vi "Capture and Playback Audio.vi"(10 "Feedback Event":refnum<user-event>, 11 "Command Queue":refnum<queue>) -> ()   [LabVIEW 2020]
uses:
  Controls/Latency Test Message.ctl
  Controls/Audio Device Refnum.ctl
  Controls/Latency Test Config.ctl
  Controls/Backends.ctl
  Controls/Latency Test Device Config.ctl
  Controls/Audio Device Config.ctl
  Controls/Audio Device Format.ctl
  Controls/Audio Device Advanced Config.ctl
  Controls/Latency Test Loopback State.ctl
  Controls/Audio Device Type.ctl
  Controls/Audio Device Info.ctl
  Controls/Audio Device Native Data Format.ctl
  888dee6f-a1d8-44b9-8463-aaa634a31580.vi
  afe3ba56-811c-4ec0-8caf-7165a7675817.vi
  Private/Result To Error.vi
  888dee6f-a1d8-44b9-8463-aaa634a31580.vi/6b901882-6109-4f44-aca5-48e1525e5248.vi
  888dee6f-a1d8-44b9-8463-aaa634a31580.vi/06c0137a-63d3-4e30-982f-115d83a1188c.vi
  Audio Devices/Get Audio Device Configuration.vi
  Private/Audio Device Refnum To Value.vi
  afe3ba56-811c-4ec0-8caf-7165a7675817.vi/4dfb5711-8d81-45a3-b3db-a84d40650863.vi
  afe3ba56-811c-4ec0-8caf-7165a7675817.vi/c8869513-30c6-44f2-a2d3-73232fe63870.vi
  888dee6f-a1d8-44b9-8463-aaa634a31580.vi/06c0137a-63d3-4e30-982f-115d83a1188c.vi/4b7b629c-2e91-4160-9820-a26af8f6e677.vi
  Private/ma_format To Audio Data Format.vi
  afe3ba56-811c-4ec0-8caf-7165a7675817.vi/4dfb5711-8d81-45a3-b3db-a84d40650863.vi/4b7b629c-2e91-4160-9820-a26af8f6e677.vi
  afe3ba56-811c-4ec0-8caf-7165a7675817.vi/c8869513-30c6-44f2-a2d3-73232fe63870.vi/4b7b629c-2e91-4160-9820-a26af8f6e677.vi
  <vilib>/Utility/Data Type/Get Numeric Information.vi
  <vilib>/Utility/error.llb/Error Cluster From Error Code.vi
  G-Audio.lvlib
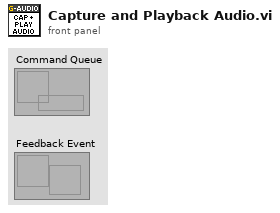
[diagram p1: front panel]
types:
  T1 = typedef "G-Audio.lvlib/Audio Device Refnum.ctl" = refnum<file>
  T2 = typedef "Latency Test Config.ctl" = cluster{"Backend":T3, "Read / Write Buffer":i32, "Capture Device":T4, "Playback Device":T4}
  T3 = typedef "G-Audio.lvlib/Backends.ctl" = enum16{"WASAPI", "DirectSound", "WinMM", "Core Audio", "sndio", "audio(4)", "OSS", "PulseAudio", "ALSA", "JACK", "AAudio", "OpenSL|ES", "Web Audio", "Custom", "Null", "Default"}
  T4 = typedef "Latency Test Device Config.ctl" = cluster{"Name":u16, "ID":u8[], "Buffer Size":u32, "Config":T5, "Advanced Config":T7}
  T5 = typedef "G-Audio.lvlib/Audio Device Config.ctl" = cluster{"Sample Rate (Hz)":u32, "Channels":u32, "Format":T6}
  T6 = typedef "G-Audio.lvlib/Audio Device Format.ctl" = enum16{"Native", "U8", "I16", "I32", "SGL"}
  T7 = typedef "G-Audio.lvlib/Audio Device Advanced Config.ctl" = cluster{"Exclusive Mode":bool, "Period Size":u32, "Num Periods":u32, "Optimize Latency":bool}
  T8 = typedef "Latency Test Loopback State.ctl" = enum16{"Idle", "Init", "Loopback", "Stop", "Shutdown", "Error"}
  T9 = typedef "Latency Test Message.ctl" = cluster{"Info":string, "Data":variant}
  T10 = typedef "G-Audio.lvlib/Audio Device Type.ctl" = enum16{"(None)", "Playback", "Capture", "Duplex", "Loopback"}
  T11 = typedef "G-Audio.lvlib/Audio Device Info.ctl" = cluster{"Name":string, "ID":u8[], "Device Type":T10, "Default":bool, "Native Data Formats":T12[]}
  T12 = typedef "G-Audio.lvlib/Audio Device Native Data Format.ctl" = cluster{"Format":T6, "Channels":u32, "Sample Rate (Hz)":u32, "Exclusive Mode":bool}
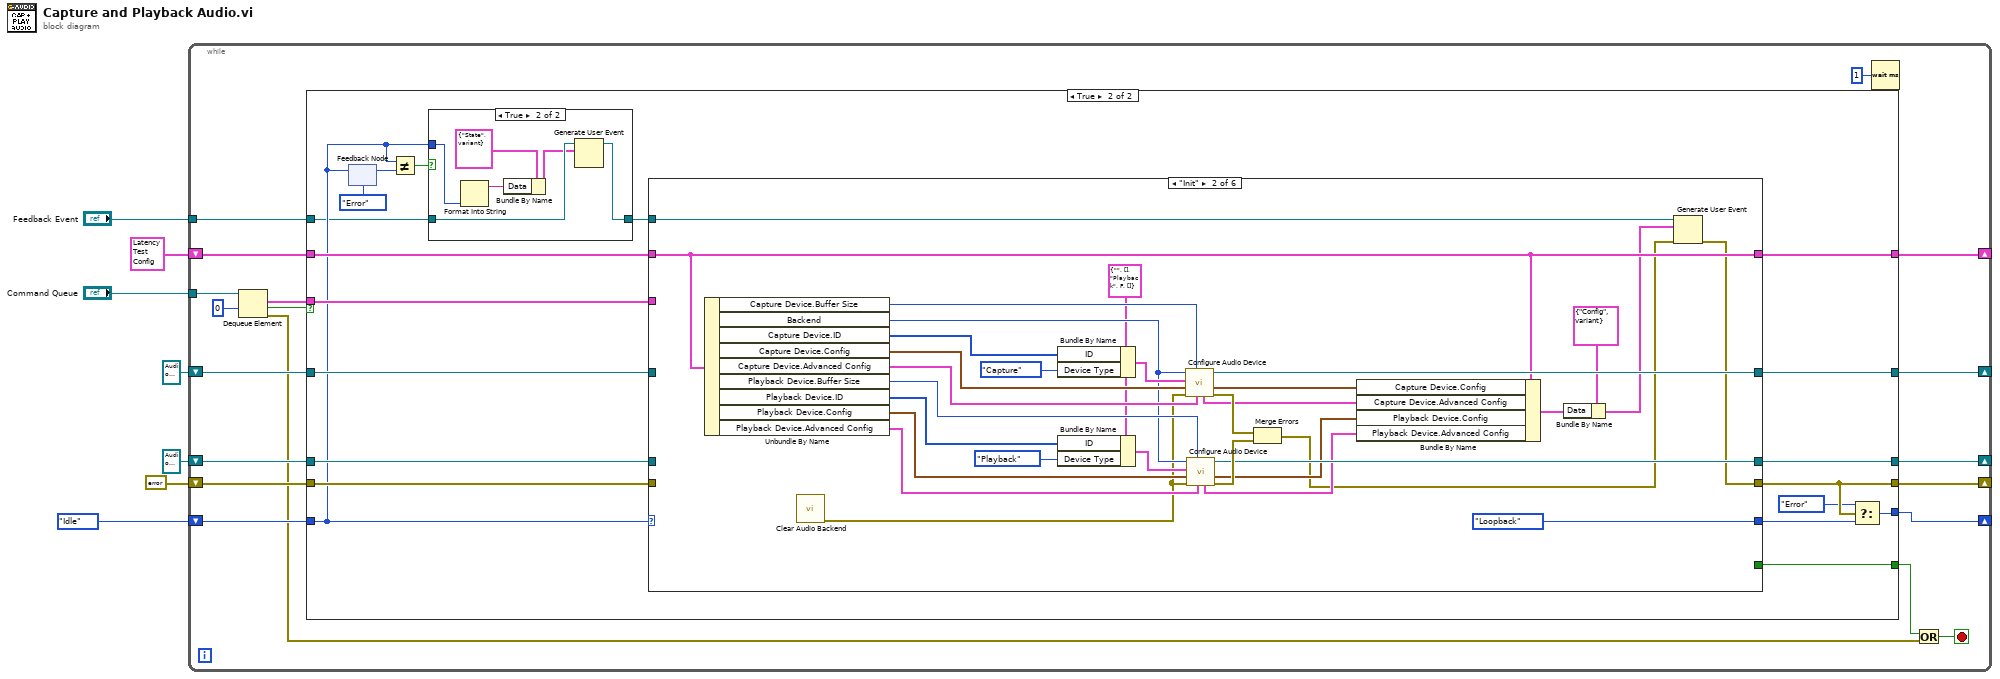
[diagram p0: block diagram]
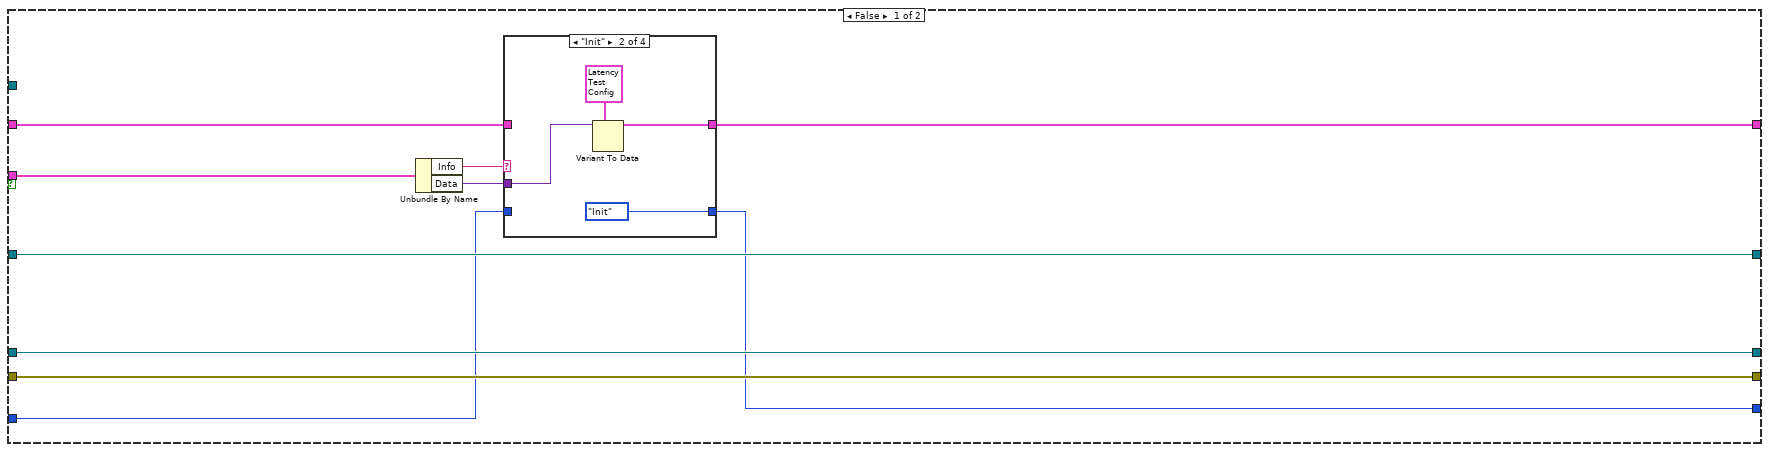
[diagram p2: hidden frame]
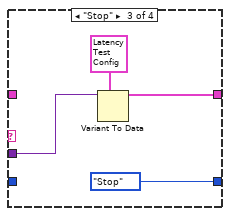
[diagram p4: hidden frame]
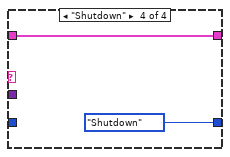
[diagram p5: hidden frame]
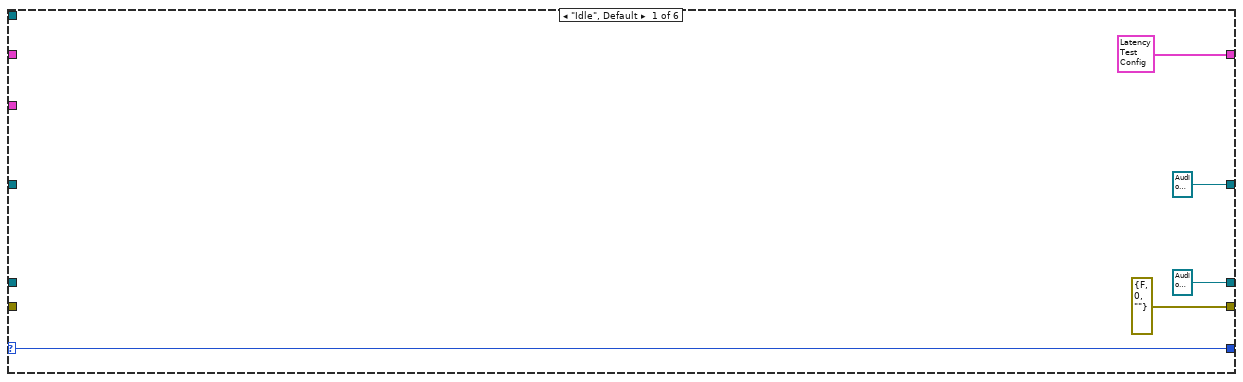
[diagram p7: hidden frame]
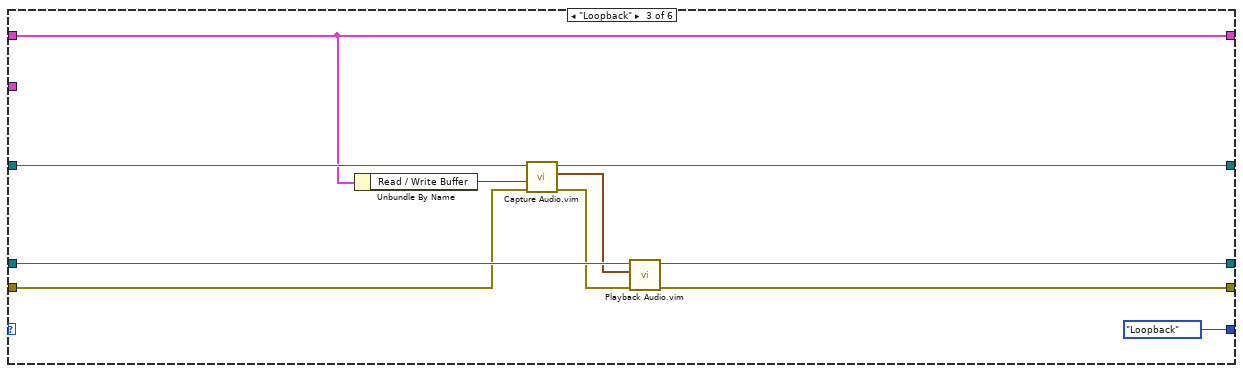
[diagram p8: hidden frame]
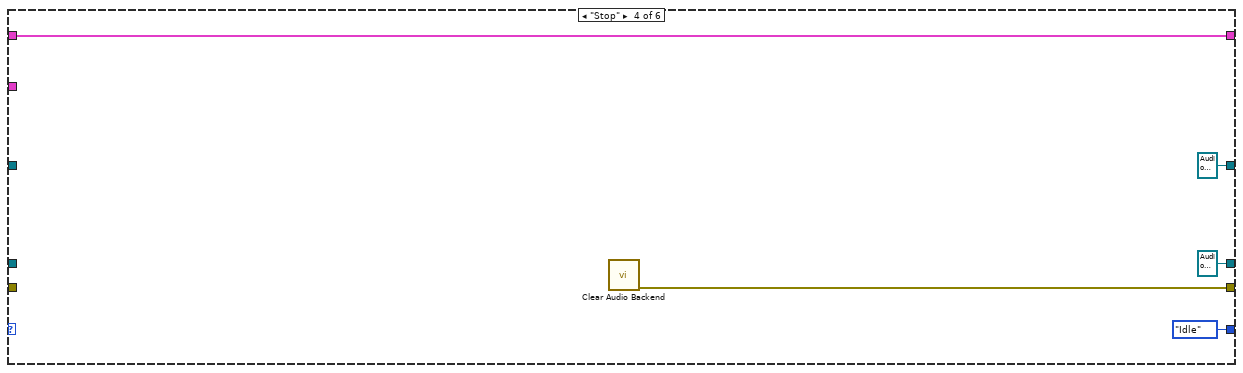
[diagram p9: hidden frame]
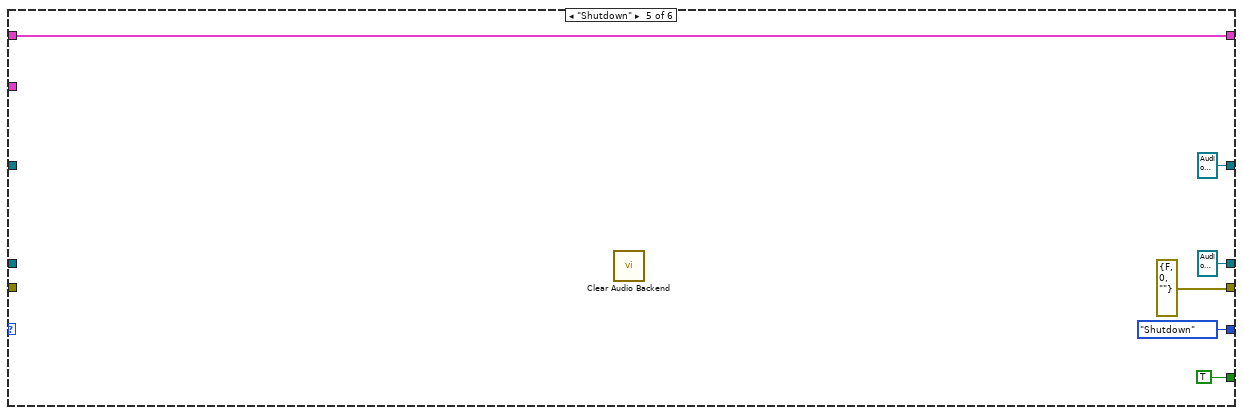
[diagram p10: hidden frame]
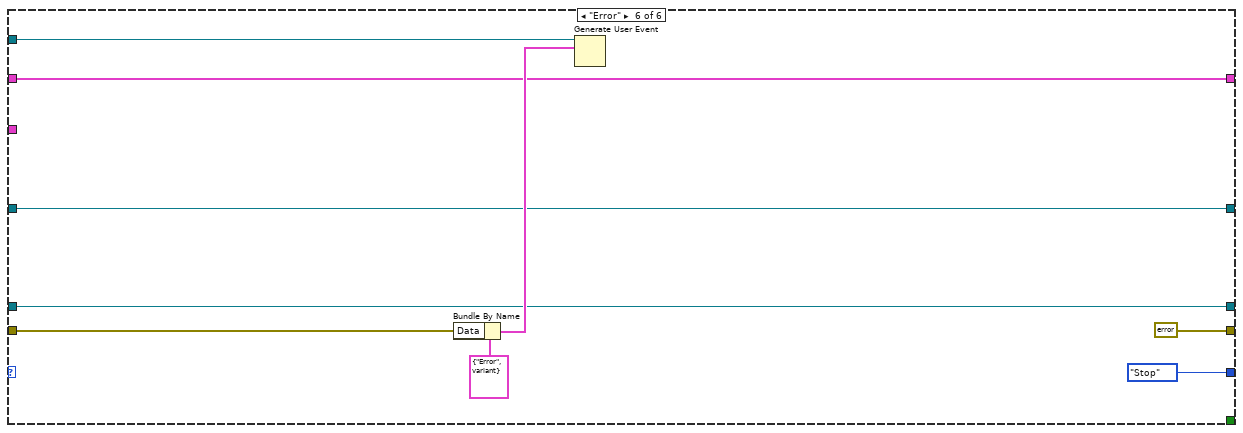
[diagram p11: hidden frame]
diagram:
  n1 = while {
    tunnel: "Command Queue" -> [w26]
    shift-right: [w21] -> _
    shift-left: Latency_Test_Loopback_State."Idle" ("Loopback State") -> [w24]
    shift-right: [w22] -> _
    shift-left: T2 {"Backend"=enum."WASAPI", "Read / Write Buffer"=0, "Capture Device"={"Name"=0, "ID"=[], "Buffer Size"=0, "Config"={"Sample Rate (Hz)"=0, "Channels"=0, "Format"=enum."Native"}, "Advanced Config"={"Exclusive Mode"=FALSE, "Period Size"=0, "Num Periods"=0, "Optimize Latency"=FALSE}}, "Playback Device"={"Name"=0, "ID"=[], "Buffer Size"=0, "Config"={"Sample Rate (Hz)"=0, "Channels"=0, "Format"=enum."Native"}, "Advanced Config"={"Exclusive Mode"=FALSE, "Period Size"=0, "Num Periods"=0, "Optimize Latency"=FALSE}}} ("Cluster") -> [w20]
    shift-right: [w17] -> _
    shift-left: errorcluster {"status"=FALSE, "code"=0, "source"=""} ("error IO") -> [w16]
    shift-right: [w15] -> _
    shift-left: T1 refnum ("Audio Device Refnum") -> [w19]
    shift-right: [w14] -> _
    shift-left: T1 refnum ("Audio Device Refnum") -> [w18]
    tunnel: "Feedback Event" -> [w13]
    stop <- w9 stop-if-true
    n2 = Dequeue Element(queue=w26, timeout in ms (-1)=0) -> (element=w23:T9, timed out?=w11:bool, error out=w8:errorcluster)  [unwired: 1 in, 1 out]
    n3 = case shown="True" w11 {
      tunnel: w24 -> [w28 w51]
      tunnel: w23 -> [w36 w67]
      tunnel: [w33 w56] -> w22
      tunnel: [w27 w61] -> w21
      tunnel: w20 -> [w32 w66]
      tunnel: w19 -> [w31 w65]
      tunnel: w18 -> [w30 w64]
      tunnel: [w29 w62] -> w17
      tunnel: w16 -> [w29 w63]
      tunnel: [w31 w58] -> w15
      tunnel: [w30 w57] -> w14
      tunnel: w13 -> [_ w50]
      tunnel: [_ w55] -> w10
      frame False {
        n4 = Unbundle By Name(w36) -> ("Info"=w35:string, "Data"=w34:variant)
        n5 = case shown="\"Init\"" w35 {
          tunnel: w34 -> [_ w42 w46 _]
          tunnel: [w38 w40 w44 w48] -> w33
          tunnel: [w37 Latency_Test_Loopback_State."Init" ("Loopback State") Latency_Test_Loopback_State."Stop" ("Loopback State") Latency_Test_Loopback_State."Shutdown" ("Loopback State")] -> w27
          tunnel: w32 -> [w38 _ _ w48]
          tunnel: w28 -> [w37 _ _ _]
          frame Default {
          }
          frame "Init" {
            n6 = Variant To Data(type=T2 {"Backend"=enum."WASAPI", "Read / Write Buffer"=0, "Capture Device"={"Name"=0, "ID"=[], "Buffer Size"=0, "Config"={"Sample Rate (Hz)"=0, "Channels"=0, "Format"=enum."Native"}, "Advanced Config"={"Exclusive Mode"=FALSE, "Period Size"=0, "Num Periods"=0, "Optimize Latency"=FALSE}}, "Playback Device"={"Name"=0, "ID"=[], "Buffer Size"=0, "Config"={"Sample Rate (Hz)"=0, "Channels"=0, "Format"=enum."Native"}, "Advanced Config"={"Exclusive Mode"=FALSE, "Period Size"=0, "Num Periods"=0, "Optimize Latency"=FALSE}}} ("Cluster"), Variant=w42) -> (data=w40:T2)  [unwired: 1 in, 1 out]
          }
          frame "Stop" {
            n7 = Variant To Data(type=T2 {"Backend"=enum."WASAPI", "Read / Write Buffer"=0, "Capture Device"={"Name"=0, "ID"=[], "Buffer Size"=0, "Config"={"Sample Rate (Hz)"=0, "Channels"=0, "Format"=enum."Native"}, "Advanced Config"={"Exclusive Mode"=FALSE, "Period Size"=0, "Num Periods"=0, "Optimize Latency"=FALSE}}, "Playback Device"={"Name"=0, "ID"=[], "Buffer Size"=0, "Config"={"Sample Rate (Hz)"=0, "Channels"=0, "Format"=enum."Native"}, "Advanced Config"={"Exclusive Mode"=FALSE, "Period Size"=0, "Num Periods"=0, "Optimize Latency"=FALSE}}} ("Cluster"), Variant=w46) -> (data=w44:T2)  [unwired: 1 in, 1 out]
          }
          frame "Shutdown" {
          }
        }
      }
      frame True {
        n8 = feedback-in #1(w51) -> ()
        n9 = feedback #1(Latency_Test_Loopback_State."Error" ("Loopback State")) -> (w53:T8)
        n10 = Not Equal?(x=w51, y=w53) -> (x != y?=w52:bool)
        n11 = case shown="True" w52 {
          tunnel: w51 -> [_ w72]
          tunnel: w50 -> [w68 w74]
          tunnel: [w68 w73] -> w49
          frame False {
          }
          frame True {
            n12 = Format Into String(w72) -> (resulting string=w70:string)  [unwired: 3 in, 1 out]
            n13 = Bundle By Name(cluster=T9 {"Info"="State", "Data"=variant} ("event data"), "Data"=w70) -> (w69:T9)
            n14 = Generate User Event(user event=w74, event data cluster=w69) -> (user event out=w73:refnum<user-event>)  [unwired: 2 in, 1 out]
          }
        }
        n15 = case shown="\"Init\"" w51 {
          selector: w51 -> [w77 _ _ _ _ _]
          tunnel: w67 -> [_ _ _ _ _ _]
          tunnel: w66 -> [_ w86 w120 w125 w131 w133]
          tunnel: w65 -> [_ _ w121 _ _ w134]
          tunnel: w64 -> [_ _ w118 _ _ w135]
          tunnel: [errorcluster {"status"=FALSE, "code"=0, "source"=""} ("error IO") w80 w113 w126 errorcluster {"status"=FALSE, "code"=0, "source"=""} ("error out") errorcluster {"status"=FALSE, "code"=0, "source"=""} ("error out")] -> w62
          tunnel: w63 -> [_ _ w114 _ _ w140]
          tunnel: [w77 Latency_Test_Loopback_State."Loopback" ("Loopback State") Latency_Test_Loopback_State."Loopback" ("Loopback State") Latency_Test_Loopback_State."Idle" ("Loopback State") Latency_Test_Loopback_State."Shutdown" ("Loopback State") Latency_Test_Loopback_State."Stop" ("Loopback State")] -> w60
          tunnel: [T1 refnum ("Audio Device Refnum") w92 w115 T1 refnum ("Audio Device Refnum Out") T1 refnum ("Audio Device Refnum Out") w134] -> w58
          tunnel: [T1 refnum ("Audio Device Refnum") w91 w117 T1 refnum ("Audio Device Refnum Out") T1 refnum ("Audio Device Refnum Out") w135] -> w57
          tunnel: [T2 {"Backend"=enum."WASAPI", "Read / Write Buffer"=0, "Capture Device"={"Name"=0, "ID"=[], "Buffer Size"=0, "Config"={"Sample Rate (Hz)"=0, "Channels"=0, "Format"=enum."Native"}, "Advanced Config"={"Exclusive Mode"=FALSE, "Period Size"=0, "Num Periods"=0, "Optimize Latency"=FALSE}}, "Playback Device"={"Name"=0, "ID"=[], "Buffer Size"=0, "Config"={"Sample Rate (Hz)"=0, "Channels"=0, "Format"=enum."Native"}, "Advanced Config"={"Exclusive Mode"=FALSE, "Period Size"=0, "Num Periods"=0, "Optimize Latency"=FALSE}}} ("Cluster") w86 w120 w125 w131 w133] -> w56
          tunnel: w49 -> [_ w85 _ _ _ w141]
          tunnel: [_ _ _ _ TRUE _] -> w55
          frame "Idle", Default {
          }
          frame "Init" {
            w99 = T11 {"Name"="", "ID"=[], "Device Type"=enum."Playback", "Default"=FALSE, "Native Data Formats"=[]} ("Audio Device")
            n16 = Unbundle By Name(w86) -> ("Capture Device.Buffer Size"=w104:u32, "Backend"=w102:T3, "Capture Device.ID"=w110:u8[], "Capture Device.Config"=w106:T5, "Capture Device.Advanced Config"=w105:T7, "Playback Device.Buffer Size"=w103:u32, "Playback Device.ID"=w101:u8[], "Playback Device.Config"=w98:T5, "Playback Device.Advanced Config"=w97:T7)
            n17 = call "Clear Audio Backend.vi"() -> ("error out"=w96:errorcluster)  [unwired: 11 in]
            n18 = Bundle By Name(cluster=w99, "ID"=w110, "Device Type"=Audio_Device_Type."Capture") -> (w108:T11)
            n19 = Bundle By Name(cluster=w99, "ID"=w101, "Device Type"=Audio_Device_Type."Playback") -> (w100:T11)
            n20 = call "Configure Audio Device.vi"("Advanced Config"=w105, "Buffer Size (4096)"=w104, "error in (no error)"=w96, "Device Config"=w106, "Audio Device"=w108, "Backend (Default)"=w102) -> ("error out"=w95:errorcluster, "Actual Device Config"=w90:T5, "Audio Device Refnum"=w92:T1, "Actual Advanced Config"=w89:T7)  [unwired: 2 in]
            n21 = call "Configure Audio Device.vi"("Advanced Config"=w97, "Buffer Size (4096)"=w103, "error in (no error)"=w96, "Device Config"=w98, "Audio Device"=w100, "Backend (Default)"=w102) -> ("error out"=w94:errorcluster, "Actual Device Config"=w88:T5, "Audio Device Refnum"=w91:T1, "Actual Advanced Config"=w87:T7)  [unwired: 2 in]
            n22 = Merge Errors(w95, w94) -> (w81:errorcluster)
            n23 = Bundle By Name(cluster=w86, "Capture Device.Config"=w90, "Capture Device.Advanced Config"=w89, "Playback Device.Config"=w88, "Playback Device.Advanced Config"=w87) -> (w83:T2)
            n24 = Bundle By Name(cluster=T9 {"Info"="Config", "Data"=variant} ("event data"), "Data"=w83) -> (w82:T9)
            n25 = Generate User Event(user event=w85, event data cluster=w82, error in=w81) -> (error out=w80:errorcluster)  [unwired: 1 in, 1 out]
          }
          frame "Loopback" {
            n26 = Unbundle By Name(w120) -> ("Read / Write Buffer"=w119:i32)
            n27 = call "Capture Audio.vim"("error in (no error)"=w114, "Samples To Read"=w119, "Audio Device Refnum In"=w121) -> ("error out"=w111:errorcluster, "Audio Data"=w112:waveform(i16)[], "Audio Device Refnum Out"=w115:T1)  [unwired: 6 in]
            n28 = call "Playback Audio.vim"("error in (no error)"=w111, "Audio Data"=w112, "Audio Device Refnum In"=w118) -> ("error out"=w113:errorcluster, "Audio Device Refnum Out"=w117:T1)  [unwired: 7 in]
          }
          frame "Stop" {
            n29 = call "Clear Audio Backend.vi"() -> ("error out"=w126:errorcluster)  [unwired: 11 in]
          }
          frame "Shutdown" {
            n30 = call "Clear Audio Backend.vi"() -> ()  [unwired: 11 in, 1 out]
          }
          frame "Error" {
            n31 = Bundle By Name(cluster=T9 {"Info"="Error", "Data"=variant} ("event data"), "Data"=w140) -> (w138:T9)
            n32 = Generate User Event(user event=w141, event data cluster=w138) -> ()  [unwired: 2 in, 2 out]
          }
        }
        n33 = Select(t=Latency_Test_Loopback_State."Error" ("Loopback State"), s=w62, f=w60) -> (s? t:f=w61:T8)
      }
    }
    n34 = Wait (ms)(milliseconds to wait=u32 1) -> ()  [unwired: 1 out]
    n35 = Or(x=w10, y=w8) -> (x .or. y?=w9:bool)
  }
